vi "GV-CursorVmove.vi"(7 "Gviewer in":refnum<class "Gviewer.lvclass">, 8 "error in (no error)":errorcluster, 9 "New coordinate":T1, 10 "Pos":cluster{"x":i16, "y":i16}, 11 "pict in":picture) -> (0 "error out":errorcluster, 3 "pict out":picture, 5 "Gviewer out":refnum<class "Gviewer.lvclass">)   [LabVIEW 2020, in "Sgraph_lib_V1.lvlib" / "Gviewer.lvclass"]
doc: "Andre Koelewijn, 30 jan 2021\n\nVertical scroll zoom cursor draw"
uses:
  Gviewer.lvclass
  <vilib>/Utility/miscctls.llb/LVPoint32TypeDef.ctl
  Gviewer.lvclass/Gviewer.ctl
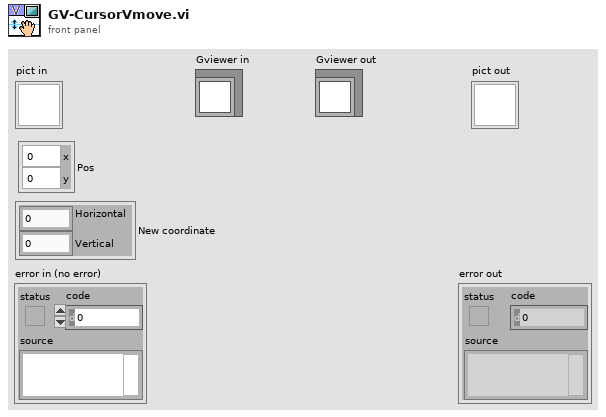
[diagram p1: front panel]
types:
  T1 = typedef "LVPoint32TypeDef.ctl" = cluster{"Horizontal":i32, "Vertical":i32}
  T2 = cluster{"horizontal":enum16{"left", "center", "right"}, "vertical":enum16{"top", "center", "bottom"}}
  T3 = cluster{"Width":u16, "Style":enum32{"Solid", "Dash", "Dot", "DashDot", "DashDotDot"}}
  T4 = typedef "Sgraph_lib_V1.lvlib/Gviewer.lvclass/Typedef_SelProperties.ctl" = cluster{"Color":u32, "LineType":T5, "max":dbl, "min":dbl}
  T5 = typedef "Sgraph_lib_V1.lvlib/Gviewer.lvclass/Typedef_LineType.ctl" = enum16{"num_bare", "num_MinMax_Area", "num_MinMax_Lines", "num_MinMax_Forfor", "num_Max_Area", "num_Max_Line", "num_Max_Forfor", "num_Min_Area", "num_Min_Line", "num_Min_Fosfor", "Boolean_Line_01", "Boolean_Area_01", "Boolean_Fosfor_01", "Boolean_Line_TF", "Boolean_Area_TF", "Boolean_Fosfor_TF", "Boolean_OnOff_Line", "Boolean_OnOff_Area", "Boolean_OnOff_Fosfor", "Boolean_spare", "StringEvent_Line", "StringEvent_TimeLine"}
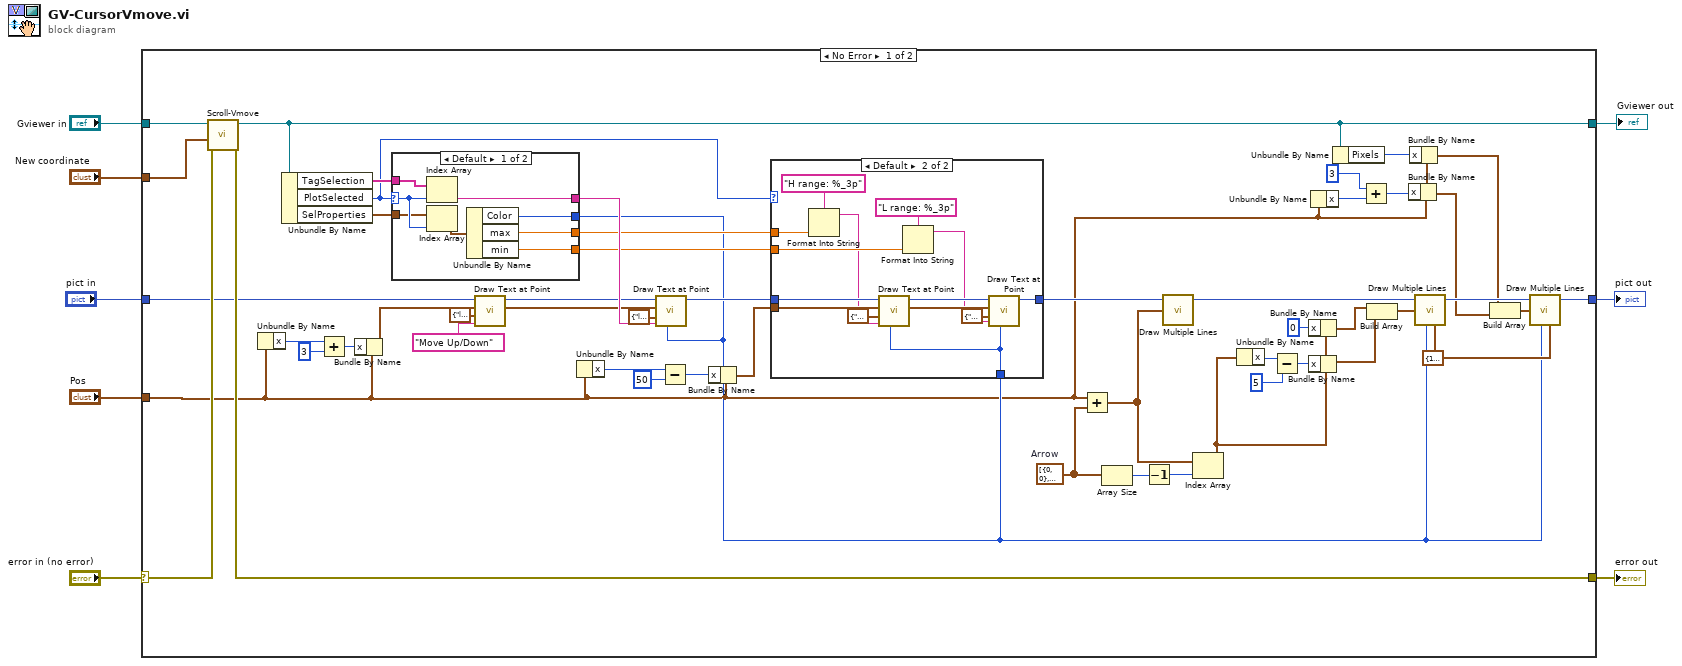
[diagram p0: block diagram]
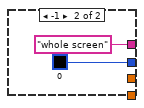
[diagram p3: hidden frame]
diagram:
  n1 = case shown="No Error" "error in (no error)" {
    selector: "error in (no error)" -> [w17 w86]
    tunnel: [w16 w86] -> w7
    tunnel: "pict in" -> [w14 w85]
    tunnel: [w44 w85] -> w5
    tunnel: "Pos" -> [w9 _]
    tunnel: "Gviewer in" -> [w19 w84]
    tunnel: [w15 w84] -> w2
    tunnel: "New coordinate" -> [w18 _]
    frame No Error {
      w53 = T3 {"Width"=1, "Style"=enum."Dash"} ("pen")
      w58 = cluster{"x":i16, "y":i16}[] [{"x"=0, "y"=0}, {"x"=-20, "y"=0}, {"x"=-20, "y"=10}, {"x"=-15, "y"=10}, {"x"=-25, "y"=20}, {"x"=-35, "y"=10}, {"x"=-30, "y"=10}, {"x"=-30, "y"=-10}, {"x"=-25, "y"=-10}, {"x"=-35, "y"=-20}, {"x"=-45, "y"=-10}, {"x"=-40, "y"=-10}, {"x"=-40, "y"=0}, {"x"=-50, "y"=0}]  # Arrow
      n2 = call "Scroll-Vmove.vi"("error in (no error)"=w17, "New coordinate"=w18, "Gviewer in"=w19) -> ("error out"=w16:errorcluster, "Gviewer out"=w15:refnum<class "Gviewer.lvclass">)  [unwired: 6 in, 1 out]
      n3 = Unbundle By Name(w9) -> ("x"=w11:i16)
      n4 = Unbundle By Name(w15) -> ("TagSelection"=w33:string[], "PlotSelected"=w20:i32, "SelProperties"=w35:T4[])
      n5 = Add(x=w11, y=i16 3) -> (x+y=w13:i16)
      n6 = Bundle By Name(cluster=w9, "x"=w13) -> (w10:cluster{"x":i16, "y":i16})
      n7 = case shown="Default" w20 {
        selector: w20 -> [w78 _]
        tunnel: w33 -> [w81 _]
        tunnel: [w74 "whole screen"] -> w34
        tunnel: w35 -> [w75 _]
        tunnel: [w79 u32 0 ("Color")] -> w21
        tunnel: [w77 _] -> w28
        tunnel: [w76 _] -> w27
        frame Default {
          n8 = Index Array(array=w81, index=w78) -> (element=w74:string)
          n9 = Index Array(array=w75, index=w78) -> (element=w80:T4)
          n10 = Unbundle By Name(w80) -> ("Color"=w79:u32, "max"=w77:dbl, "min"=w76:dbl)
        }
        frame -1 {
        }
      }
      n11 = call <vilib>:"Draw Text at Point.vi"("text"="Move Up/Down", "alignment(left, top)"=T2 {"horizontal"=enum."left", "vertical"=enum."bottom"}, "origin"=w10, "picture"=w14) -> ("new picture"=w31:picture)  [unwired: 6 in, 1 out]
      n12 = Unbundle By Name(w9) -> ("x"=w25:i16)
      n13 = call <vilib>:"Draw Text at Point.vi"("text color(black)"=w21, "text"=w34, "alignment(left, top)"=T2 {"horizontal"=enum."left", "vertical"=enum."top"}, "origin"=w10, "picture"=w31) -> ("new picture"=w29:picture)  [unwired: 5 in, 1 out]
      n14 = Subtract(x=w25, y=i16 50) -> (x-y=w23:i16)
      n15 = Bundle By Name(cluster=w9, "x"=w23) -> (w22:cluster{"x":i16, "y":i16})
      n16 = case shown="Default" w20 {
        tunnel: w29 -> [w60 w72]
        tunnel: w28 -> [_ w68]
        tunnel: w27 -> [_ w67]
        tunnel: [w60 w69] -> w26
        tunnel: w22 -> [_ w66]
        tunnel: w21 -> [_ w61]
        frame -1 {
        }
        frame Default {
          n17 = Format Into String(format string="H range: %_3p", w68) -> (resulting string=w62:string)  [unwired: 2 in, 1 out]
          n18 = call <vilib>:"Draw Text at Point.vi"("text color(black)"=w61, "text"=w62, "alignment(left, top)"=T2 {"horizontal"=enum."right", "vertical"=enum."bottom"}, "origin"=w66, "picture"=w72) -> ("new picture"=w70:picture)  [unwired: 5 in, 1 out]
          n19 = Format Into String(format string="L range: %_3p", w67) -> (resulting string=w63:string)  [unwired: 2 in, 1 out]
          n20 = call <vilib>:"Draw Text at Point.vi"("text color(black)"=w61, "text"=w63, "alignment(left, top)"=T2 {"horizontal"=enum."right", "vertical"=enum."top"}, "origin"=w66, "picture"=w70) -> ("new picture"=w69:picture)  [unwired: 5 in, 1 out]
        }
      }
      n21 = Add(x=w9, y=w58) -> (x+y=w55:cluster{"x":i16, "y":i16}[])
      n22 = Array Size(array=w58) -> (size(s)=w57:i32)
      n23 = Decrement(x=w57) -> (x-1=w56:i32)
      n24 = call <vilib>:"Draw Multiple Lines.vi"("picture"=w26, "line endpoints"=w55) -> ("new picture"=w59:picture)  [unwired: 7 in]
      n25 = Index Array(array=w55, index=w56) -> (element=w47:cluster{"x":i16, "y":i16})
      n26 = Unbundle By Name(w47) -> ("x"=w52:i16)
      n27 = Subtract(x=w52, y=i16 5) -> (x-y=w50:i16)
      n28 = Bundle By Name(cluster=w47, "x"=i16 0) -> (w46:cluster{"x":i16, "y":i16})
      n29 = Bundle By Name(cluster=w47, "x"=w50) -> (w49:cluster{"x":i16, "y":i16})
      n30 = Unbundle By Name(w9) -> ("x"=w43:i16)
      n31 = Unbundle By Name(w15) -> ("Pixels"=w30:i32)
      n32 = Add(x=i16 3, y=w43) -> (x+y=w42:i16)
      n33 = Build Array(w46, w49) -> (w54:cluster{"x":i16, "y":i16}[])
      n34 = Bundle By Name(cluster=w9, "x"=w42) -> (w39:cluster{"x":i16, "y":i16})
      n35 = Bundle By Name(cluster=w9, "x"=w30) -> (w38:cluster{"x":i16, "y":i16})
      n36 = call <vilib>:"Draw Multiple Lines.vi"("picture"=w59, "line endpoints"=w54, "color(black)"=w21, "pen"=w53) -> ("new picture"=w45:picture)  [unwired: 5 in]
      n37 = Build Array(w38, w39) -> (w40:cluster{"x":i16, "y":i16}[])
      n38 = call <vilib>:"Draw Multiple Lines.vi"("picture"=w45, "line endpoints"=w40, "color(black)"=w21, "pen"=w53) -> ("new picture"=w44:picture)  [unwired: 5 in]
    }
    frame Error {
    }
  }
  "error out" <- w7
  "pict out" <- w5
  "Gviewer out" <- w2
